vi "Release Queue and Notifier.vi"(8 "error in (no error)":errorcluster, 10 "Queue and Notifier":T1, 11 "Instrument.DAQ in":refnum<class "Instrument.DAQ.lvclass">) -> (0 "error out":errorcluster, 3 "Instrument.DAQ out":refnum<class "Instrument.DAQ.lvclass">)   [LabVIEW 2019, in "Instrument.Lockin.lvlib" / "Instrument.DAQ.lvclass"]
uses:
  Instrument.DAQ.lvclass
  Typedefs/Queue and Notifier.ctl
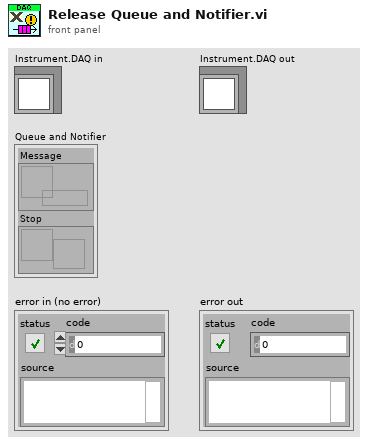
[diagram p1: front panel]
types:
  T1 = typedef "Instrument.Lockin.lvlib/Instrument.DAQ.lvclass/Queue and Notifier.ctl" = cluster{"Message":refnum<queue>, "Stop":refnum<notifier>}
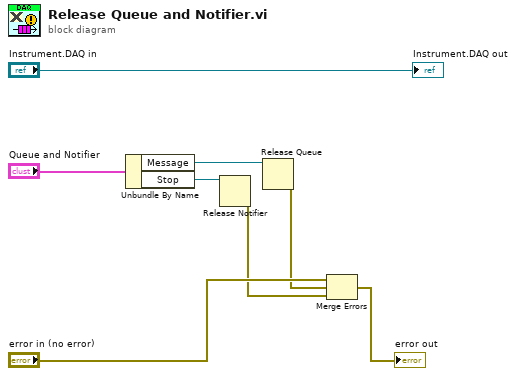
[diagram p0: block diagram]
diagram:
  n1 = Unbundle By Name("Queue and Notifier") -> ("Message"=w5:refnum<queue>, "Stop"=w6:refnum<notifier>)
  n2 = Release Notifier(notifier=w6) -> (error out=w2:errorcluster)  [unwired: 2 in, 2 out]
  n3 = Release Queue(queue=w5) -> (error out=w3:errorcluster)  [unwired: 2 in, 2 out]
  n4 = Merge Errors("error in (no error)", w3, w2) -> (→"error out":errorcluster)
  "Instrument.DAQ out" <- "Instrument.DAQ in"
